vi "Set WIFI Security Type.vi"(8 "Error In":errorcluster, 10 "WIFI Security Type":T1=enum."WPA2 Password", 11 "LINX Device Config":T2) -> (0 "Error Out":errorcluster, 3 "LINX Device Config":T2)   [LabVIEW 2020, in "Device.lvlib"]
doc: "Set the LINX device's WIFI Security Type."
uses:
  Device.lvlib
  Type Defs/Error Type.ctl
  LMH-LINX.lvlib
  Type Defs/Interface.ctl
  Type Defs/WIFI Security Type.ctl
  Type Defs/Channels.ctl
  Type Defs/TCP Config.ctl
  Type Defs/LINX Device Config.ctl
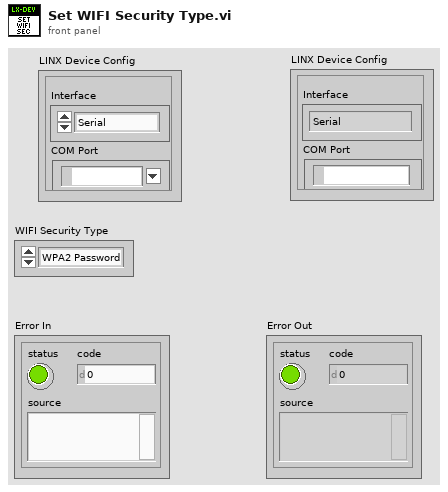
[diagram p1: front panel]
types:
  T1 = typedef "LMH-LINX.lvlib/WIFI Security Type.ctl" = enum8{"None", "WPA2 Password", "WPA2 Key", "WEP40", "WEP104"}
  T2 = typedef "Device.lvlib/LINX Device Config.ctl" = cluster{"Interface":T3, "COM Port":refnum<visa-resource-name>, "TCP Configuration":T4, "Device Family":u8, "Device ID":u8, "Device Name":string, "TCP Ref":refnum<k5>, "Channels":T5}
  T3 = typedef "LMH-LINX.lvlib/Interface.ctl" = enum16{"Serial", "TCP"}
  T4 = typedef "Device.lvlib/TCP Config.ctl" = cluster{"IP Address":string, "Port":u16}
  T5 = typedef "LMH-LINX.lvlib/Channels.ctl" = cluster{"DI":u8[], "DO":u8[], "AI":u8[], "AO":u8[], "PWM":u8[], "QE":u8[], "UART":u8[], "I2C 2":u8[], "SPI":u8[], "CAN":u8[], "Servo":u8[], "AI Ref (V)":dbl, "AI Resolution (Bits)":u8, "AO Ref (V)":dbl, "AO Resolution (Bits)":u8}
  T6 = typedef "LMH-LINX.lvlib/Error Type.ctl" = enum16{"Unknown", "Timeout", "Corrupt Return Packet", "Unable To Connect", "Command Not Supported", "Channel DNE", "Invalid COM Config", "Firmware Version Mismatch", "myRIO Support", "CMD Specific Error", "Local IO Not Supported"}
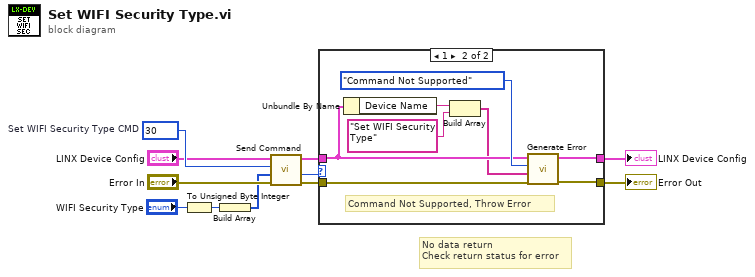
[diagram p0: block diagram]
diagram:
  w10 = u16 30  # Set WIFI Security Type CMD
  # "No data return\nCheck return status for error"
  n1 = To Unsigned Byte Integer(number="WIFI Security Type") -> (unsigned 8bit integer=w1:u8)
  n2 = Build Array(w1) -> (w3:u8[])
  n3 = call "Send Command.vi"("Error In"="Error In", "ARGS"=w3, "CMD"=w10, "LINX Device Config"="LINX Device Config") -> ("Error Out"=w5:errorcluster, "Status"=w4:u8, "LINX Device Config"=w7:T2)  [unwired: 4 in, 1 out]
  n4 = case shown="1" w4 {
    tunnel: [w12 w19] -> w8
    tunnel: w7 -> [w12 w15]
    tunnel: [w13 w20] -> w6
    tunnel: w5 -> [w13 w21]
    frame 0, Default {
      # "Status OK, Process Data"
    }
    frame 1 {
      # "Command Not Supported, Throw Error"
      n5 = Unbundle By Name(w15) -> ("Device Name"=w16:string)
      n6 = Build Array(w16, "Set WIFI Security Type") -> (w14:string[])
      n7 = call "Generate Error.vi"("Error In"=w21, "Arguments"=w14, "Error Type"=Error_Type."Command Not Supported", "LINX Device Config"=w15) -> ("Error Out"=w20:errorcluster, "Dup LINX Device Config"=w19:T2)  [unwired: 6 in]
    }
  }
  "Error Out" <- w6
  "LINX Device Config" <- w8
